vi "ToString.vi"(1 "Request":refnum<class "Request.lvclass">) -> (0 "String":string)   [LabVIEW 2023, in "Request.lvclass"]
doc: "Format/Serialize this Request to a uniquely identifying string."
uses:
  Request.lvclass
  Get Request.vi
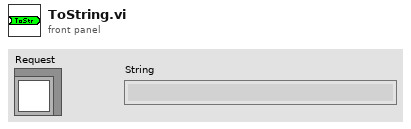
[diagram p1: front panel]
types:
  T1 = typedef "Request.ctl" = cluster{"Method":string, "URI":string, "Protocol":string, "Raw Path":string, "Query":string, "Fragment":string, "Raw Body":string, "Headers":variant, "Parameters":variant, "Body":variant, "Raw Header":string, "Path":string[]}
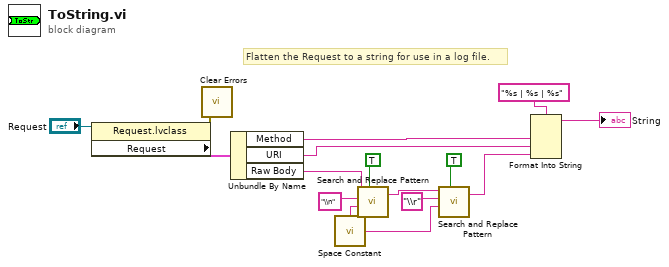
[diagram p0: block diagram]
diagram:
  # "Flatten the Request to a string for use in a log file."
  n1 = property on="Property Node" class="Request.lvclass"(reference="Request") -> (error out=w12:errorcluster, "Request"=w11:T1)  [unwired: 1 in, 1 out]
  n2 = call <vilib>:"Clear Errors.vi"("error in (no error)"=w12) -> ()  [unwired: 5 in, 2 out]
  n3 = Unbundle By Name(w11) -> ("Method"=w10:string, "URI"=w9:string, "Raw Body"=w8:string)
  n4 = call <vilib>:"Space Constant.vi"() -> ("String"=w1:string)
  n5 = call <vilib>:"Search and Replace Pattern.vi"("string"=w8, "regular expression (\"\")"="\\n" ("regular expression (\"\")"), "replace string (\"\")"=w1, "replace all? (F)"=TRUE) -> ("result string"=w3:string)  [unwired: 1 in, 1 out]
  n6 = call <vilib>:"Search and Replace Pattern.vi"("string"=w3, "regular expression (\"\")"="\\r" ("regular expression (\"\")"), "replace string (\"\")"=w1, "replace all? (F)"=TRUE) -> ("result string"=w2:string)  [unwired: 1 in, 1 out]
  n7 = Format Into String(format string="%s | %s | %s", w10, w9, w2) -> (resulting string=→"String":string)  [unwired: 2 in, 1 out]
